vi "Get Block List.vi"(8 "error in (no error)":errorcluster, 9 "Blob":string, 10 "Container":string, 11 "Azure Session in":refnum<class "Session.lvclass">) -> (0 "error out":errorcluster, 1 "Uncommitted Blocks":string[](array[string]), 2 "Committed Blocks":string[](array[string]), 3 "Azure Session out":refnum<class "Session.lvclass">)   [LabVIEW 2015, in "NI_Azure_Blob.lvlib"]
doc: "Retrieves the list of blocks that have been uploaded as part of a block blob."
uses:
  NI_Azure_Blob.lvlib
  Core/Session/Session.lvclass
  Core/Name Value Pair.ctl
  Core/Session/Session.lvclass/Session.ctl
  Core/Session/Write Request Parameters.vi
  Core/Session/Write HTTP Verb.vi
  Core/Session/Write URL Suffix.vi
  Core/NI_Azure_Core.lvlib
  XML Parsing/NI_Azure_XML Parsing.lvlib
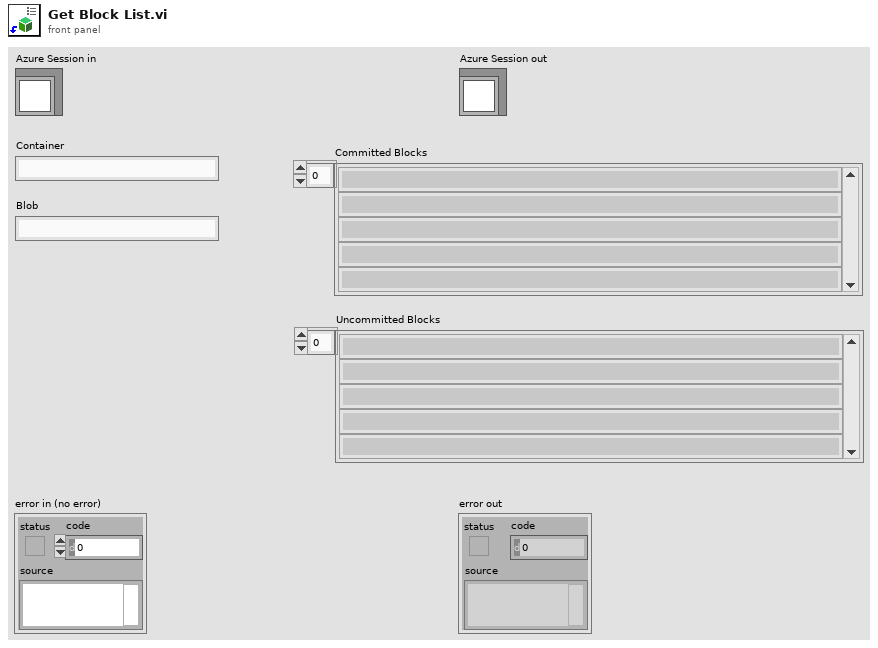
[diagram p1: front panel]
types:
  T1 = typedef "NI_Azure_Core.lvlib/Name Value Pair.ctl" = cluster{"name":string, "value":string}
  T2 = typedef "NI_Azure_Core.lvlib/Response.ctl" = cluster{"Headers":string, "Body":string}
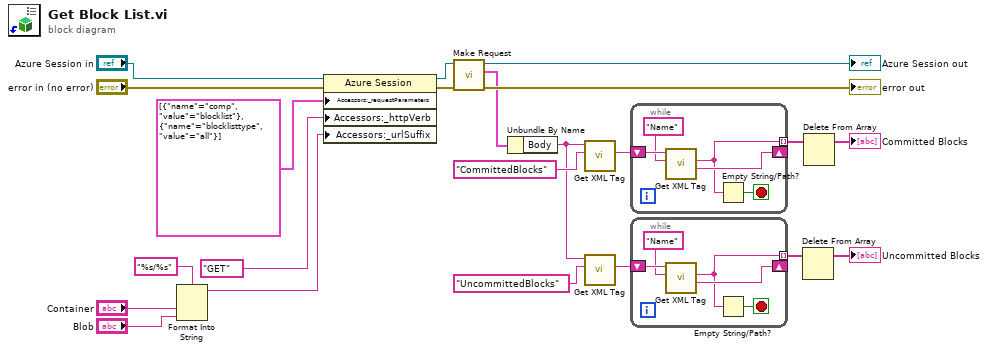
[diagram p0: block diagram]
diagram:
  n1 = Format Into String(format string="%s/%s", "Container", "Blob") -> (resulting string=w12:string)  [unwired: 2 in, 1 out]
  n2 = property class="Azure Session"(reference="Azure Session in", error in="error in (no error)", "Accessors:_requestParameters"=T1[] [{"name"="comp", "value"="blocklist"}, {"name"="blocklisttype", "value"="all"}] ("appended array"), "Accessors:_httpVerb"="GET" ("HTTP-Verb"), "Accessors:_urlSuffix"=w12) -> (reference out=w16:refnum<class "Session.lvclass">, error out=w14:errorcluster)
  n3 = call "Make Request.vi"("error in (no error)"=w14, "Session in"=w16) -> ("error out"=→"error out":errorcluster, "Response"=w11:T2, "Session out"=→"Azure Session out":refnum<class "Session.lvclass">)  [unwired: 7 in]
  n4 = Unbundle By Name(w11) -> ("Body"=w6:string)
  n5 = call "Get XML Tag.vi"("Tag name"="CommittedBlocks", "XML String in"=w6) -> ("Tag value"=w10:string)  [unwired: 5 in, 4 out]
  n6 = call "Get XML Tag.vi"("Tag name"="UncommittedBlocks", "XML String in"=w6) -> ("Tag value"=w7:string)  [unwired: 5 in, 4 out]
  n7 = while {
    shift-right: [w26] -> _
    shift-left: w10 -> [w27]
    tunnel: [w24] -> w4 mode=indexing
    stop <- w23 stop-if-true
    n8 = call "Get XML Tag.vi"("Tag name"="Name", "XML String in"=w27) -> ("Remaining string"=w26:string, "Tag value"=w24:string)  [unwired: 5 in, 3 out]
    n9 = Empty String/Path?(string/path=w24) -> (empty?=w23:bool)
  }
  n10 = while {
    shift-right: [w31] -> _
    shift-left: w7 -> [w32]
    tunnel: [w29] -> w2 mode=indexing
    stop <- w28 stop-if-true
    n11 = call "Get XML Tag.vi"("Tag name"="Name", "XML String in"=w32) -> ("Remaining string"=w31:string, "Tag value"=w29:string)  [unwired: 5 in, 3 out]
    n12 = Empty String/Path?(string/path=w29) -> (empty?=w28:bool)
  }
  n13 = Delete From Array(array=w2) -> (array with subset deleted=→"Uncommitted Blocks":string[])  [unwired: 2 in, 1 out]
  n14 = Delete From Array(array=w4) -> (array with subset deleted=→"Committed Blocks":string[])  [unwired: 2 in, 1 out]
